vi "Set Active Slider.vi"(3 "Slider Ref":refnum<vi>, 5 "Color Ref":refnum<vi>, 6 "Ex Active Slider ID":i32, 7 "Numeric Ref":refnum<vi>, 8 "error in (no error)":errorcluster, 9 "Numeric Ref Array":refnum<vi>[](array[refnum]), 10 "Color Ref Array":refnum<vi>[](array[refnum]), 11 "Slider Ref Array":refnum<vi>[](array[refnum])) -> (0 "error out":errorcluster, 4 "New Active Slider ID":i32)   [LabVIEW 2020, in "3D Plot.lvclass"]
uses:
  <vilib>/Math Plots/3D Math Plots/3D Plot/3D Plot/3D Plot.lvclass
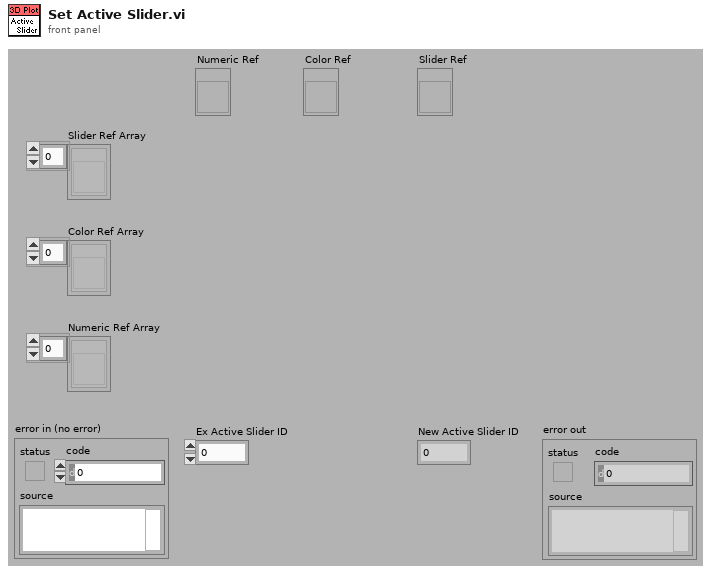
[diagram p1: front panel]
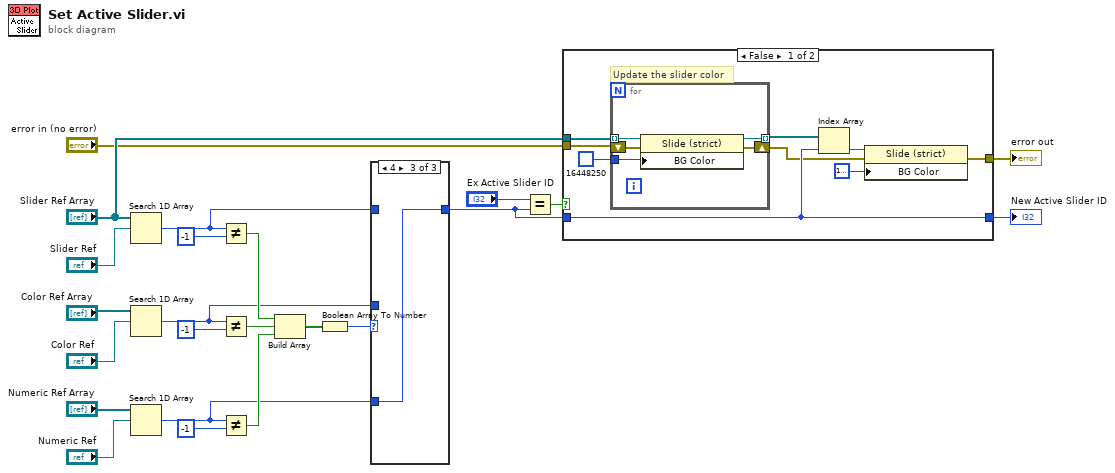
[diagram p0: block diagram]
diagram:
  n1 = Search 1D Array(1D array="Slider Ref Array", element="Slider Ref") -> (index of element=w10:i32)  [unwired: 1 out]
  n2 = Search 1D Array(1D array="Color Ref Array", element="Color Ref") -> (index of element=w9:i32)  [unwired: 1 out]
  n3 = Search 1D Array(1D array="Numeric Ref Array", element="Numeric Ref") -> (index of element=w8:i32)  [unwired: 1 out]
  n4 = Not Equal?(x=w10, y=-1) -> (x != y?=w15:bool)
  n5 = Not Equal?(x=w9, y=-1) -> (x != y?=w14:bool)
  n6 = Not Equal?(x=w8, y=-1) -> (x != y?=w13:bool)
  n7 = Build Array(w15, w14, w13) -> (w12:bool[])
  n8 = Boolean Array To Number(Boolean array=w12) -> (number=w11:u32)
  n9 = case shown="4" w11 {
    tunnel: [w24 w25 w26] -> w4
    tunnel: w10 -> [w24 _ _]
    tunnel: w9 -> [_ w25 _]
    tunnel: w8 -> [_ _ w26]
    frame 1, Default {
    }
    frame 2 {
    }
    frame 4 {
    }
  }
  n10 = Equal?(x="Ex Active Slider ID", y=w4) -> (x = y?=w6:bool)
  n11 = case shown="False" w6 {
    tunnel: "Slider Ref Array" -> [w32 _]
    tunnel: w4 -> [w30 w42]
    tunnel: [w30 w42] -> w3
    tunnel: "error in (no error)" -> [w29 w41]
    tunnel: [w27 w41] -> w1
    frame False {
      # "Update the slider color"
      n12 = for {
        tunnel: [w39] -> w31 mode=indexing
        tunnel: w32 -> [w40] mode=indexing
        tunnel: u32 16448250 -> [w38]
        shift-right: [w36] -> w28
        shift-left: w29 -> [w37]
        n13 = property class="Slide (strict)"(reference=w40, error in=w37, "BG Color"=w38) -> (reference out=w39:refnum<vi>, error out=w36:errorcluster)
      }
      n14 = Index Array(array=w31, index=w30) -> (element=w35:refnum<vi>)
      n15 = property class="Slide (strict)"(reference=w35, error in=w28, "BG Color"=u32 16777222) -> (error out=w27:errorcluster)  [unwired: 1 out]
    }
    frame True {
    }
  }
  "New Active Slider ID" <- w3
  "error out" <- w1
